vi "UpdateMathematicaImage.vi"(11 "Mathematica Settings":T1) -> ()   [LabVIEW 2017]
uses:
  MathematicaSettingsCtl.ctl
  controls/GlobalExp.vi
  Global.lvlib
panel:
  out "standard error":string
  out "standard output":string
  out "command":string
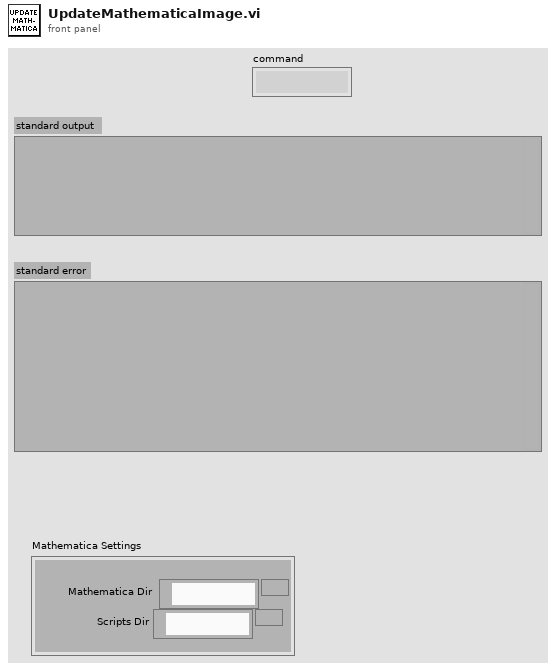
[diagram p1: front panel]
types:
  T1 = typedef "MathematicaSettingsCtl.ctl" = cluster{"Mathematica Dir":path, "Scripts Dir":path}
  T2 = typedef "MasterExpControl.ctl" = cluster{"Main Steps":dbl, "Main Runs":dbl, "ExpStatus":enum16{"Innit", "Stop", "Idle", "MainRunning", "AuxRunning"}, "Main Current Step":dbl, "ExpNum":dbl, "NewData":bool, "date":string, "command":string, "Stop":bool, "Pause":bool, "Mathematica":string, "Main/Meta":bool, "UpdateMath":bool, "Camera":bool}
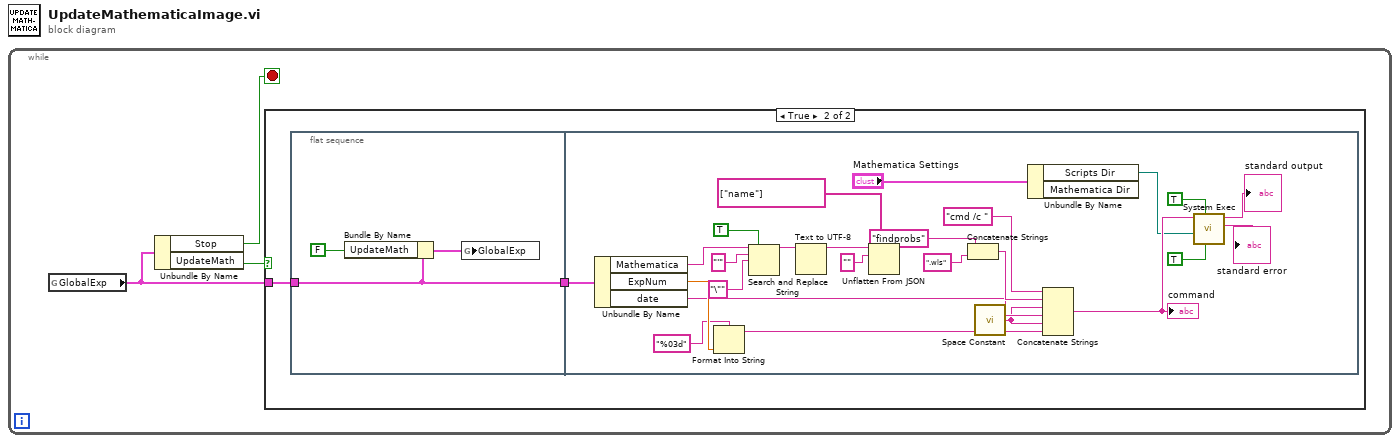
[diagram p0: block diagram]
diagram:
  n1 = while {
    stop <- w1 stop-if-true
    n2 = global read "GlobalExp.vi" "GlobalExp"() -> (w2:T2)
    n3 = Unbundle By Name(w2) -> ("Stop"=w1:bool, "UpdateMath"=w3:bool)
    n4 = case shown="True" w3 {
      tunnel: w2 -> [_ w5]
      frame False {
      }
      frame True {
        n5 = flat-sequence {
          tunnel: w5 -> [w6]
          tunnel: [w6] -> w4
          tunnel: w4 -> [w19]
          frame #0 {
            n6 = Bundle By Name(cluster=w6, "UpdateMath"=FALSE) -> (w8:T2)
            n7 = global write "GlobalExp.vi" "GlobalExp"(w8) -> ()
          }
          frame #1 {
            n8 = Unbundle By Name(w19) -> ("Mathematica"=w29:string, "ExpNum"=w22:dbl, "date"=w16:string)
            n9 = Format Into String(format string="%03d", w22) -> (resulting string=w14:string)  [unwired: 2 in, 1 out]
            n10 = Search and Replace String(replace all?=TRUE ("replace all? (F)"), input string=w29, search string="'", replace string="\"" ("replace string (\"\")")) -> (result string=w20:string)  [unwired: 4 in, 3 out]
            n11 = Text to UTF-8(11:w20) -> (3:w33:string)  [unwired: 2 in, 1 out]
            n12 = Unflatten From JSON(path=string[] ["name"], JSON string=w33, type and defaults="") -> ()  [unwired: 4 in, 2 out]
            n13 = Concatenate Strings("findprobs" ("string"), ".wls" ("string")) -> (w17:string)
            n14 = call <vilib>:"Space Constant.vi"() -> ("String"=w15:string)
            n15 = Unbundle By Name("Mathematica Settings") -> ("Scripts Dir"=w18:path)  [unwired: 1 out]
            n16 = Concatenate Strings("cmd /c ", w17, w15, w16, w15, w14) -> (w25:string)
            "command" <- w25
            n17 = call <vilib>:"System Exec.vi"("run minimized? (F)"=TRUE, "wait until completion? (T)"=TRUE, "working directory"=w18, "command line"=w25) -> ("standard error"=→"standard error":string, "standard output"=→"standard output":string)  [unwired: 4 in, 2 out]
          }
        }
      }
    }
  }
